vi "Enqueue Message.vi"(6 "Priority Message? (F)":bool, 7 "timeout in ms (-1)":i32, 8 "error in (no error)":errorcluster, 9 "Message Data":variant, 10 "Message":string, 11 "Queue":refnum<queue>) -> (0 "error out":errorcluster, 3 "Queue out":refnum<queue>)   [LabVIEW 2013]
doc: "For a regular message, enqueue the message. For a priority message, enqueue it at the front of the queue."
uses:
  Typedefs/Message Cluster.ctl
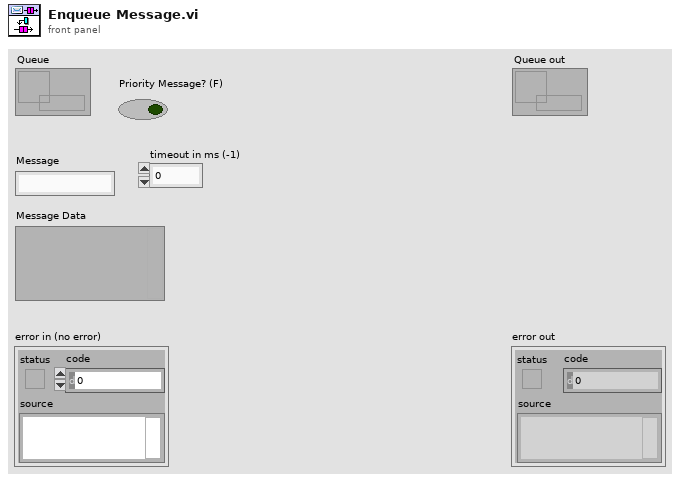
[diagram p1: front panel]
types:
  T1 = typedef "Message Cluster.ctl" = cluster{"Message":string, "Message Data":variant}
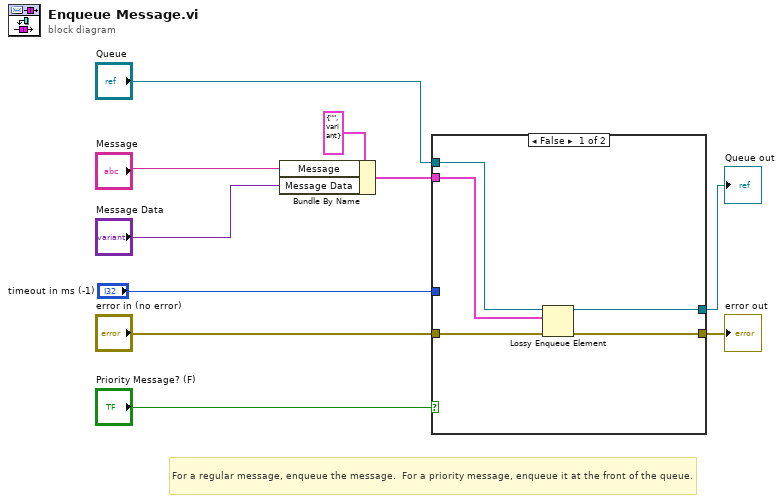
[diagram p0: block diagram]
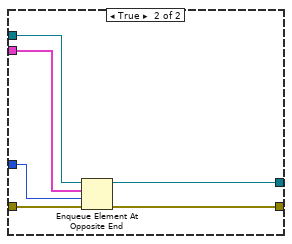
[diagram p2: hidden frame]
diagram:
  # "For a regular message, enqueue the message.  For a priority message, enqueue it at the front of the queue."
  n1 = Bundle By Name(cluster=T1 {"Message"="", "Message Data"=variant} ("Message Cluster"), "Message"="Message", "Message Data"="Message Data") -> (w4:T1)
  n2 = case shown="False" "Priority Message? (F)" {
    tunnel: "error in (no error)" -> [w15 w21]
    tunnel: [w14 w20] -> w5
    tunnel: "Queue" -> [w13 w19]
    tunnel: w4 -> [w12 w18]
    tunnel: [w11 w17] -> w2
    tunnel: "timeout in ms (-1)" -> [_ w16]
    frame False {
      n3 = Lossy Enqueue Element(queue=w13, element=w12, error in (no error)=w15) -> (queue out=w11:refnum<queue>, error out=w14:errorcluster)  [unwired: 2 out]
    }
    frame True {
      n4 = Enqueue Element At Opposite End(queue=w19, element=w18, timeout in ms (-1)=w16, error in (no error)=w21) -> (queue out=w17:refnum<queue>, error out=w20:errorcluster)  [unwired: 1 out]
    }
  }
  "error out" <- w5
  "Queue out" <- w2
